vi "Save Specific DAC Cfg Template.vi"(8 "error in":errorcluster, 10 "Default Config File Refnum":T1, 11 "DAC in":refnum<class "DAC.lvclass">) -> (0 "error out":errorcluster, 2 "refnum out":T1, 3 "DAC out":refnum<class "DAC.lvclass">)   [LabVIEW 2019, in "DAC.lvlib" / "DAC.lvclass"]
uses:
  DAC.lvclass
  <vilib>/Utility/config.llb/Config Data RefNum.ctl
  DAC.lvclass/DAC.ctl
  <vilib>/Utility/config.llb/Write Key (String).vi
  <vilib>/Utility/config.llb/Write Key (Double).vi
  <vilib>/Utility/config.llb/NI_LVConfig.lvlib
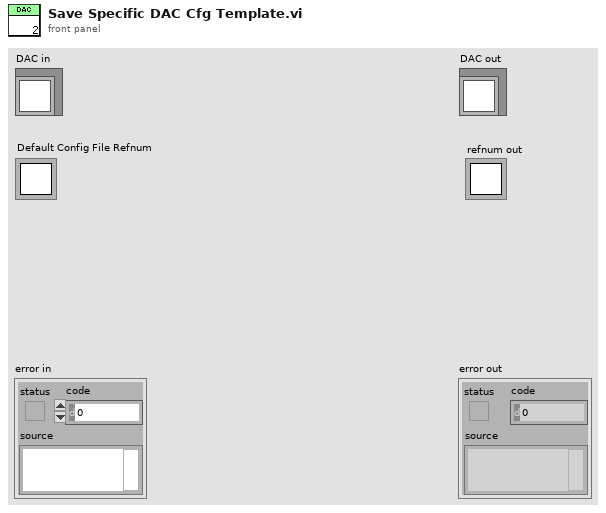
[diagram p1: front panel]
types:
  T1 = typedef "NI_LVConfig.lvlib/Config Data RefNum.ctl" = refnum<k1>
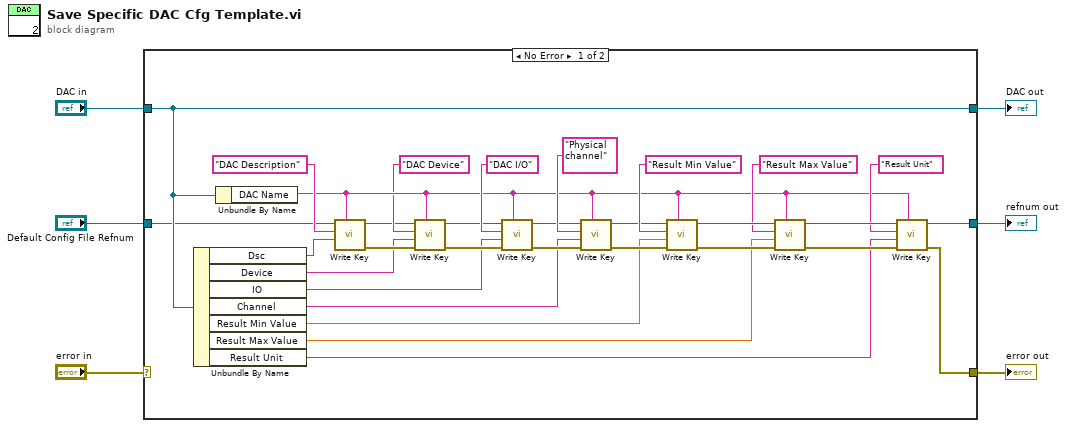
[diagram p0: block diagram]
diagram:
  n1 = case shown="No Error" "error in" {
    selector: "error in" -> [_ w40]
    tunnel: [w7 w40] -> w5
    tunnel: [w35 w39] -> w3
    tunnel: "DAC in" -> [w35 w39]
    tunnel: "Default Config File Refnum" -> [w21 w38]
    tunnel: [w8 w38] -> w1
    frame No Error {
      n2 = Unbundle By Name(w35) -> ("Dsc"=w36:string, "Device"=w14:string, "IO"=w13:string, "Channel"=w12:string, "Result Min Value"=w11:dbl, "Result Max Value"=w10:dbl, "Result Unit"=w9:string)
      n3 = Unbundle By Name(w35) -> ("DAC Name"=w20:string)
      n4 = call-poly <vilib>:"Write Key.vi"("section"=w20, "value"=w36, "key"="DAC Description", "refnum"=w21) -> ("error out"=w16:errorcluster, "refnum out"=w18:T1)  [unwired: 5 in, 1 out]
      n5 = call-poly <vilib>:"Write Key.vi"("section"=w20, "error in (no error)"=w16, "value"=w14, "key"="DAC Device", "refnum"=w18) -> ("error out"=w15:errorcluster, "refnum out"=w17:T1)  [unwired: 4 in, 1 out]
      n6 = call-poly <vilib>:"Write Key.vi"("section"=w20, "error in (no error)"=w15, "value"=w13, "key"="DAC I/O", "refnum"=w17) -> ("error out"=w23:errorcluster, "refnum out"=w24:T1)  [unwired: 4 in, 1 out]
      n7 = call-poly <vilib>:"Write Key.vi"("section"=w20, "error in (no error)"=w23, "value"=w12, "key"="Physical channel", "refnum"=w24) -> ("error out"=w26:errorcluster, "refnum out"=w27:T1)  [unwired: 4 in, 1 out]
      n8 = call-poly <vilib>:"Write Key.vi"("section"=w20, "error in (no error)"=w26, "value"=w11, "key"="Result Min Value", "refnum"=w27) -> ("error out"=w32:errorcluster, "refnum out"=w34:T1)  [unwired: 4 in, 1 out]
      n9 = call-poly <vilib>:"Write Key.vi"("section"=w20, "error in (no error)"=w32, "value"=w10, "key"="Result Max Value", "refnum"=w34) -> ("error out"=w31:errorcluster, "refnum out"=w33:T1)  [unwired: 4 in, 1 out]
      n10 = call-poly <vilib>:"Write Key.vi"("section"=w20, "error in (no error)"=w31, "value"=w9, "key"="Result Unit", "refnum"=w33) -> ("error out"=w7:errorcluster, "refnum out"=w8:T1)  [unwired: 4 in, 1 out]
    }
    frame Error {
    }
  }
  "error out" <- w5
  "DAC out" <- w3
  "refnum out" <- w1
